vi "Set Actor Name.vi"(8 "error in (no error)":errorcluster, 9 "Actor_name":string, 11 "Parent in":refnum<class "Parent_Class.lvclass">=refnum) -> (0 "error out":errorcluster, 1 "Actor_Name":string, 3 "Parent out":refnum<class "Parent_Class.lvclass">)   [LabVIEW 2023]
uses:
  Parent_Class.lvclass
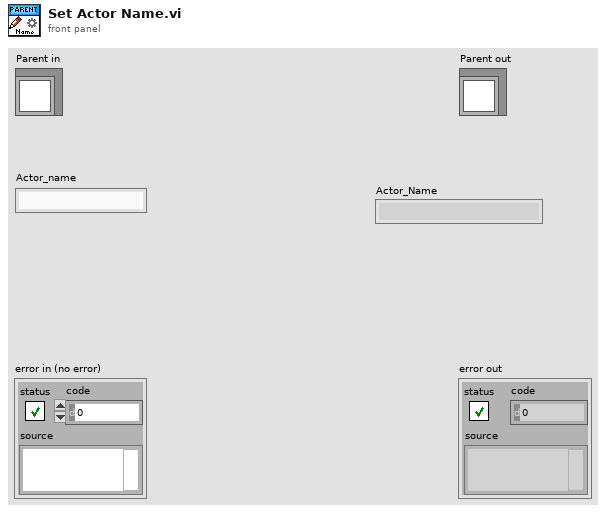
[diagram p1: front panel]
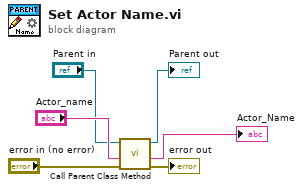
[diagram p0: block diagram]
diagram:
  n1 = call-parent "Call Parent Class Method"("error in (no error)"="error in (no error)", "Actor_name"="Actor_name", "Interface_Class in"="Parent in") -> ("error out"=→"error out":errorcluster, "Actor_Name"=→"Actor_Name":string, "Interface_Class out"=→"Parent out":refnum<class "Parent_Class.lvclass">)  [unwired: 6 in]
